vi "Retrieve Taus.vi"(8 "error in":errorcluster, 11 "CRDS Cell in":refnum<class "CRDS Cell.lvclass">) -> (0 "error out":errorcluster, 2 "Request Restart?":bool, 3 "CRDS Cell out":refnum<class "CRDS Cell.lvclass">)   [LabVIEW 2018, in "CRDS Lib.lvlib" / "CRDS Cell.lvclass"]
doc: "Takes the ringdown data for the cell acquired over a 1 s period and retrieves the averaged tau based on the average of the shot fits. This VI will also populate the statistics in the extinction cluster and provide both a decimated trace and a decimated trace for the fit using the A, B and tau parameters retrieved.\n\nAll math is linear - no errors are thrown except potentially in accessors for CRDS data."
uses:
  CRDS Cell.lvclass
  CRDS Cell.lvclass/CRDS Cell.ctl
  Data/Cell/CRDS Cell Data.lvclass/CRDS Cell Data.ctl
  General/Math/Fit Exponential Class/Fit Exponential.lvclass/Fit Exponential.ctl
  <vilib>/Analysis/baseanly.llb/Mean (DBL).vi
  General/Math/Fit Exponential Class/Read Output.vi
  General/Math/Fit Exponential Class/Get Dt.vi
  Data/Cell/Write Laser Data.vi
  Data/Cell/Read extParam.vi
  Data/Cell/Write extParam.vi
  Data/Cell/Write Allan Variances.vi
  Data/Cell/Write taus.vi
  Data/Cell/Write Ringdowns.vi
  <vilib>/Analysis/NI_AALBase.lvlib
  General/Math Utilities.lvlib
  General/Math/Fit Exponential Class/Fit Exponential.lvclass
  Data/Cell/CRDS Cell Data.lvclass
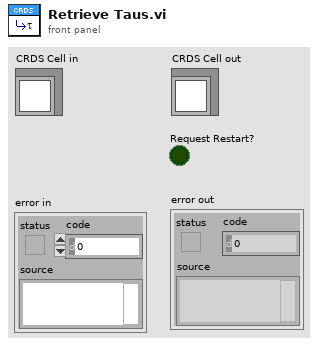
[diagram p1: front panel]
types:
  T1 = typedef "CRDS Lib.lvlib/CRDS Cell Data.lvclass/extParam Ctl.ctl" = cluster{"Tau":sgl, "Tau0cor":sgl, "ext":sgl, "extCorr":sgl, "stdevTau":sgl, "eTau":sgl, "taucorr":sgl, "Tau0":sgl, "max":sgl}
  T2 = cluster{"A":dbl, "B":dbl, "tau":dbl, "e_tau":dbl}
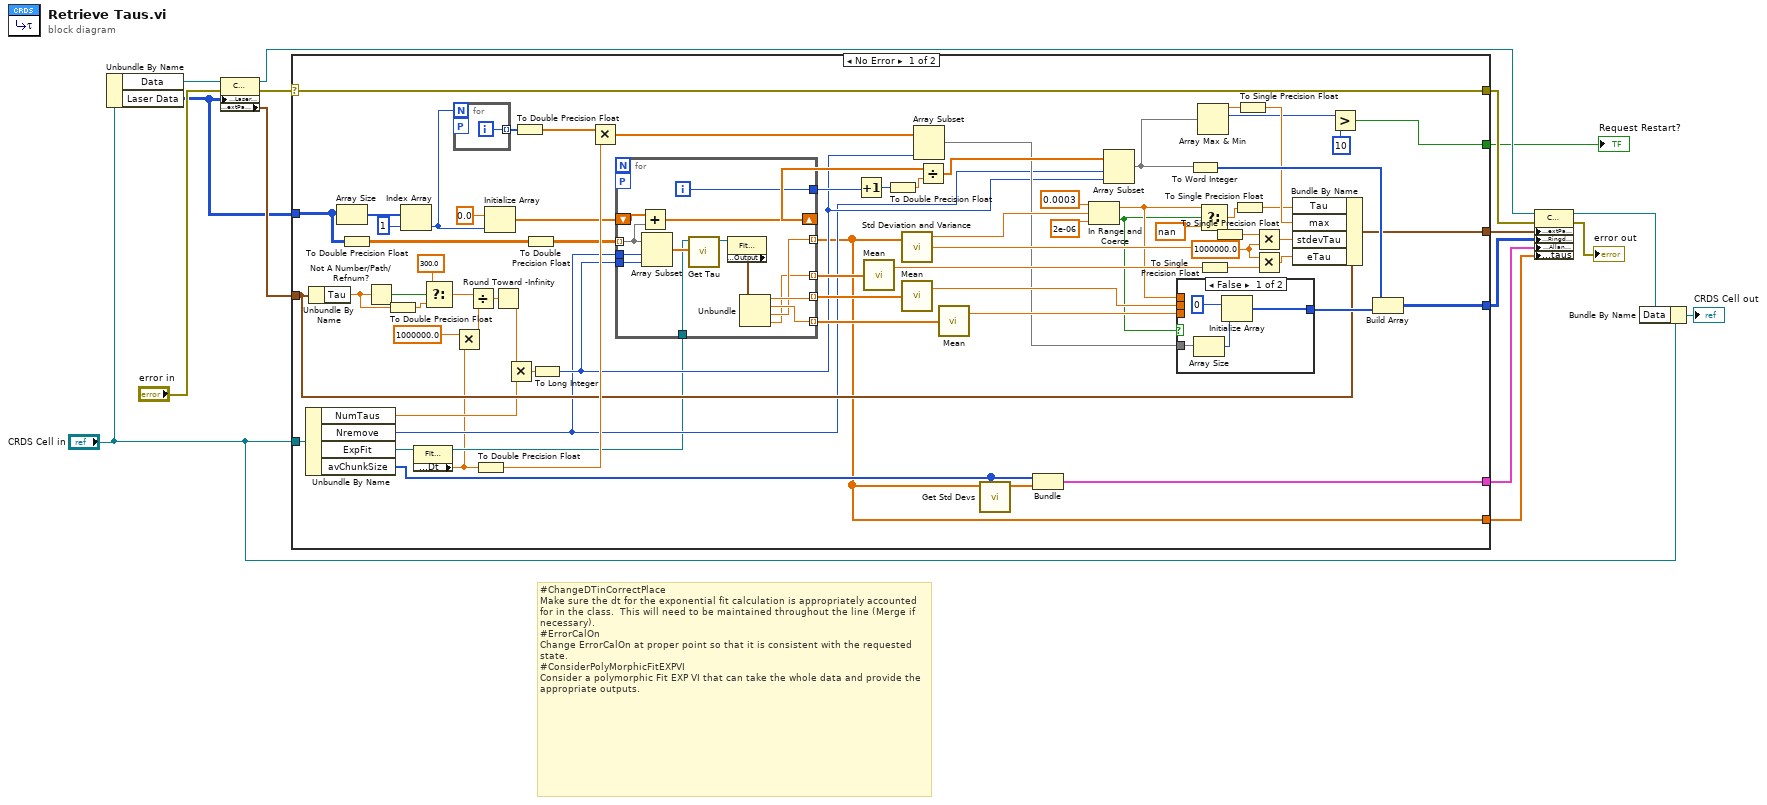
[diagram p0: block diagram]
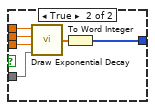
[diagram p2: hidden frame]
diagram:
  # "#ChangeDTinCorrectPlace\nMake sure the dt for the exponential fit calculation is appropriately accounted for in the class.  This will need to be maintained throughout the line (Merge if necessary).\n#ErrorCalOn\nChange ErrorCalOn at proper point so that it is consistent with the requested state.\n#ConsiderPolyMorphicFitEXPVI\nConsider a polymorphic Fit EXP VI that can take the whole data and provide the appropriate outputs."
  n1 = Unbundle By Name("CRDS Cell in") -> ("Data"=w10:refnum<class "CRDS Cell Data.lvclass">, "Laser Data"=w2:i16[][])
  n2 = property class="CRDS Cell"(reference=w10, error in="error in", "Accessors:Laser Data"=w2) -> (reference out=w11:refnum<class "CRDS Cell Data.lvclass">, error out=w12:errorcluster, "Data Access:extParam"=w3:T1)
  n3 = case shown="No Error" w12 {
    selector: w12 -> [w42 w114]
    tunnel: [w42 w114] -> w15
    tunnel: "CRDS Cell in" -> [w41 _]
    tunnel: w3 -> [w56 w113]
    tunnel: [w57 _] -> w7
    tunnel: [w52 w113] -> w16
    tunnel: [w34 _] -> w6
    tunnel: [w20 _] -> w5
    tunnel: [w18 _] -> w4
    tunnel: w2 -> [w17 _]
    frame No Error {
      w45 = sgl 1000000.0
      n4 = Unbundle By Name(w41) -> ("NumTaus"=w36:sgl, "Nremove"=w25:i32, "ExpFit"=w24:refnum<class "Fit Exponential.lvclass">, "avChunkSize"=w19:i32[])
      n5 = Unbundle By Name(w56) -> ("Tau"=w40:sgl)
      n6 = Array Size(array=w17) -> (size(s)=w72:i32[])
      n7 = To Double Precision Float(number=w17) -> (double precision float=w38:dbl[][])
      n8 = Not A Number/Path/Refnum?(number/path/refnum=w40) -> (NaN/Path/Refnum?=w61:bool)
      n9 = To Double Precision Float(number=w40) -> (double precision float=w39:dbl)
      n10 = Index Array(array=w72, index=1) -> (element=w58:i32)
      n11 = property class="Fit Exp"(reference=w24) -> (reference out=w23:refnum<class "Fit Exponential.lvclass">, "Accessors:Dt"=w22:dbl)  [unwired: 1 in, 1 out]
      n12 = Select(t=300.0, s=w61, f=w39) -> (s? t:f=w59:dbl)
      n13 = for {
        N: w58 -> [_]
        tunnel: [w112] -> w76 mode=indexing
        workers-P: _ -> [_]
        i -> [w112]
      }
      n14 = Multiply(x=1000000.0, y=w22) -> (x*y=w47:dbl)
      n15 = Divide(x=w59, y=w47) -> (x/y=w70:dbl)
      n16 = To Double Precision Float(number=w22) -> (double precision float=w86:dbl)
      n17 = Initialize Array(0.0 ("element"), w58) -> (w66:dbl[])
      n18 = Round Toward -Infinity(1:w70) -> (0:w79:dbl)
      n19 = Multiply(x=w79, y=w36) -> (x*y=w83:dbl)
      n20 = To Double Precision Float(number=w76) -> (double precision float=w75:dbl[])
      n21 = To Double Precision Float(number=w38) -> (double precision float=w37:dbl[][])
      n22 = To Long Integer(number=w83) -> (32bit integer=w26:i32)
      n23 = Multiply(x=w75, y=w86) -> (x*y=w50:dbl[])
      n24 = for {
        tunnel: [w99] -> w18 mode=indexing
        tunnel: w37 -> [w109] mode=indexing
        tunnel: [w98] -> w62 mode=indexing
        tunnel: [w101] -> w63 mode=indexing
        tunnel: [w100] -> w64 mode=indexing
        shift-right: [w111] -> w67
        shift-left: w66 -> [w110]
        tunnel: [w106] -> w74
        tunnel: w26 -> [w108]
        tunnel: w25 -> [w107]
        tunnel: w23 -> [w104]
        workers-P: _ -> [_]
        i -> [w106]
        n25 = Add(x=w110, y=w109) -> (x+y=w111:dbl[])
        n26 = Array Subset(array=w109, index=w107, length=w108) -> (w105:dbl[])
        n27 = call "Get Tau.vi"("Data In"=w105, "Fit Exp in"=w104) -> ("Fit Exp out"=w103:refnum<class "Fit Exponential.lvclass">)  [unwired: 8 in, 1 out]
        n28 = property class="Fit Exp"(reference=w103) -> ("Accessors:Output"=w102:T2)  [unwired: 1 in, 2 out]
        n29 = Unbundle(w102) -> ("A"=w101:dbl, "B"=w100:dbl, "tau"=w99:dbl, "e_tau"=w98:dbl)
      }
      n30 = Increment(x=w74) -> (x+1=w81:i32)
      n31 = call-poly <vilib>:"Mean.vi"("X"=w62) -> ("mean"=w77:dbl)  [unwired: 1 out]
      n32 = To Double Precision Float(number=w81) -> (double precision float=w80:dbl)
      n33 = call <vilib>:"Std Deviation and Variance.vi"("X"=w18) -> ("mean"=w71:dbl, "standard deviation"=w78:dbl)  [unwired: 1 in, 1 out]
      n34 = call-poly <vilib>:"Mean.vi"("X"=w63) -> ("mean"=w68:dbl)  [unwired: 1 out]
      n35 = Array Subset(array=w50, length=w26) -> (w49:dbl[])  [unwired: 1 in]
      n36 = Divide ("mean")(x=w67, y=w80) -> (x/y=w51:dbl[])
      n37 = call-poly <vilib>:"Mean.vi"("X"=w64) -> ("mean"=w69:dbl)  [unwired: 1 out]
      n38 = call "Get Std Devs.vi"("ChunkSize"=w19, "DataIn"=w18) -> ("StdDevOut"=w21:sgl[])  [unwired: 9 in]
      n39 = Bundle("avChunkSize"=w19, "StdDevOut"=w21) -> (w20:cluster{"avChunkSize":i32[], "StdDevOut":sgl[]})  [unwired: 1 in]
      n40 = In Range and Coerce(upper limit=0.0003, x=w71, lower limit=2e-06) -> (coerced(x)=w30:dbl, In Range?=w27:bool)
      n41 = Array Subset(array=w51, index=w25, length=w26) -> (w43:dbl[])
      n42 = case shown="False" w27 {
        tunnel: [w88 w97] -> w85
        tunnel: w69 -> [_ w96]
        tunnel: w68 -> [_ w95]
        tunnel: w49 -> [w90 w94]
        tunnel: w30 -> [_ w92]
        frame False {
          n43 = Array Size(array=w90) -> (size(s)=w89:i32)
          n44 = Initialize Array(i16 0, w89) -> (w88:i16[])
        }
        frame True {
          n45 = call "Draw Exponential Decay.vi"("time"=w94, "B"=w96, "A"=w95, "tau"=w92) -> ("ExponentialOut"=w93:dbl[])
          n46 = To Word Integer(number=w93) -> (16bit integer=w97:i16[])
        }
      }
      n47 = To Word Integer(number=w43) -> (16bit integer=w84:i16[])
      n48 = Array Max & Min(array=w43) -> (max value=w87:dbl, max index (indices)=w33:i32)  [unwired: 2 out]
      n49 = Select(t=w30, s=w27, f=nan) -> (s? t:f=w28:dbl)
      n50 = To Single Precision Float(number=w77) -> (single precision float=w82:sgl)
      n51 = To Single Precision Float(number=w78) -> (single precision float=w46:sgl)
      n52 = To Single Precision Float(number=w28) -> (single precision float=w44:sgl)
      n53 = To Single Precision Float(number=w87) -> (single precision float=w55:sgl)
      n54 = Multiply(x=w46, y=w45) -> (x*y=w54:sgl)
      n55 = Multiply(x=w45, y=w82) -> (x*y=w53:sgl)
      n56 = Bundle By Name(cluster=w56, "Tau"=w44, "max"=w55, "stdevTau"=w54, "eTau"=w53) -> (w52:T1)
      n57 = Greater?(x=w33, y=10) -> (0:w34:bool)
      n58 = Build Array(w84, w85) -> (w57:i16[][])
    }
    frame Error {
    }
  }
  "Request Restart?" <- w6
  n59 = property class="CRDS Cell"(reference=w11, error in=w15, "Data Access:extParam"=w16, "Data Access:Ringdowns"=w7, "Data Access:Allan Variances"=w5, "Accessors:taus"=w4) -> (reference out=w9:refnum<class "CRDS Cell Data.lvclass">, error out=→"error out":errorcluster)
  n60 = Bundle By Name(cluster="CRDS Cell in", "Data"=w9) -> (→"CRDS Cell out":refnum<class "CRDS Cell.lvclass">)
